vi "AI RT FIFO (by ref).vi"(0 "Data IN":dbl[](array[numeric]), 1 "Mode":T1=enum."Delete", 7 "Buffer Size":i32=10, 9 "# of elements":i32=1, 11 "Error IN":errorcluster, 12 "System Index":i32) -> (4 "Data OUT":dbl[][](array[numeric]), 6 "Empty?":bool, 8 "Size":i32, 15 "Error OUT":errorcluster)   [LabVIEW 2023]
uses:
  Type Defs and Controls/RT FIFO Mode.ctl
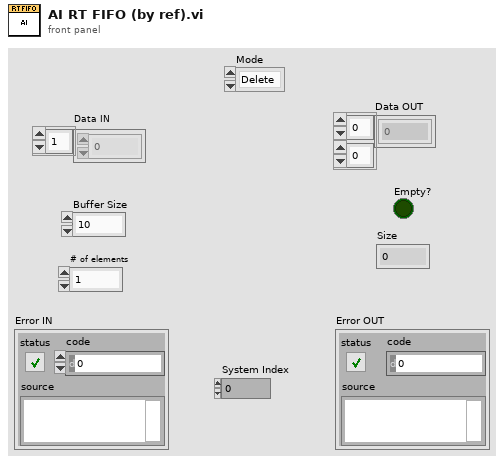
[diagram p1: front panel]
types:
  T1 = typedef "RT FIFO Mode.ctl" = enum16{"Create", "Write", "Read", "Delete"}
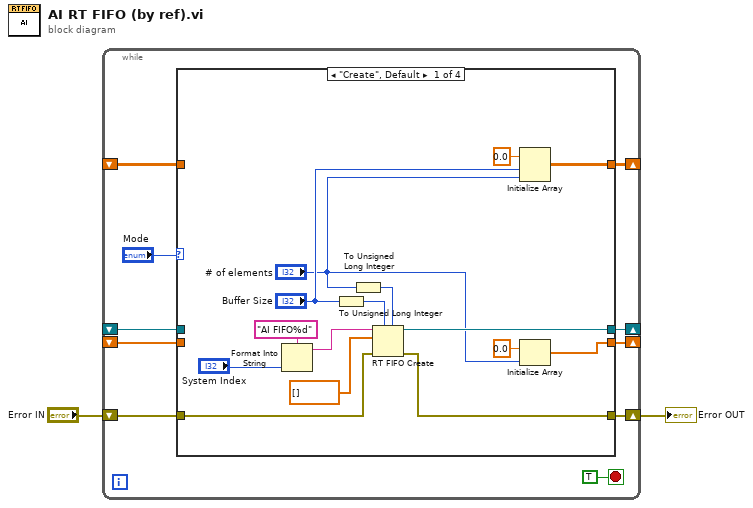
[diagram p0: block diagram]
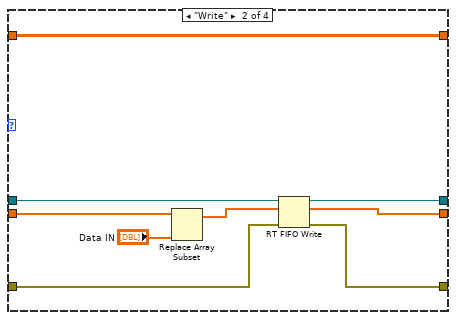
[diagram p2: hidden frame]
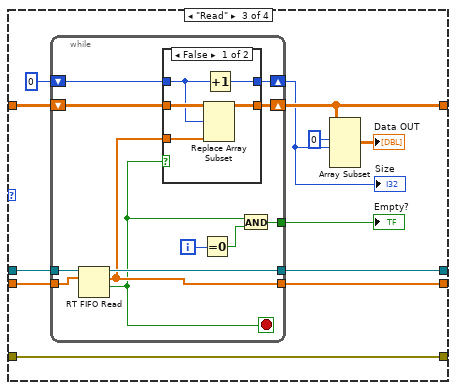
[diagram p3: hidden frame]
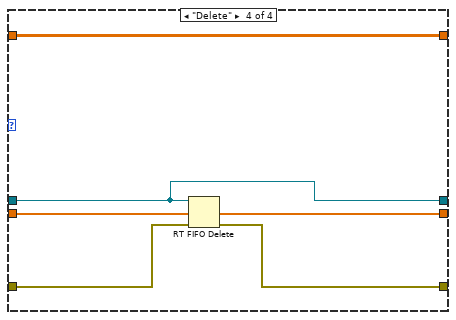
[diagram p5: hidden frame]
diagram:
  n1 = while {
    shift-right: [w10] -> _
    shift-left: _ -> [w9]
    shift-right: [w6] -> _
    shift-left: _ -> [w5]
    shift-right: [w4] -> _
    shift-left: _ -> [w3]
    shift-right: [w7] -> w1
    shift-left: "Error IN" -> [w8]
    stop <- TRUE stop-if-true
    n2 = case shown="\"Create\", Default" "Mode" {
      tunnel: [w27 w34 w45 w71] -> w10
      tunnel: w9 -> [_ w35 w46 w71]
      tunnel: w8 -> [w23 w30 w47 w69]
      tunnel: [w22 w29 w47 w68] -> w7
      tunnel: [w24 w31 w43 w70] -> w6
      tunnel: w5 -> [_ w33 w44 w70]
      tunnel: [w16 w28 w40 w67] -> w4
      tunnel: w3 -> [_ w28 w41 w67]
      frame "Create", Default {
        n3 = Format Into String(format string="AI FIFO%d" ("name (unnamed)"), "System Index") -> (resulting string=w13:string)  [unwired: 2 in, 1 out]
        n4 = To Unsigned Long Integer(number="Buffer Size") -> (unsigned 32bit integer=w17:u32)
        n5 = To Unsigned Long Integer(number="# of elements") -> (unsigned 32bit integer=w21:u32)
        n6 = RT FIFO Create(0:w13, 1:dbl[] [], 3:w23, 4:w17, 6:w21) -> (8:w27:refnum<k33>, 11:w22:errorcluster)  [unwired: 3 in, 1 out]
        n7 = Initialize Array(0.0, "Buffer Size", "# of elements") -> (w16:dbl[][])
        n8 = Initialize Array(0.0, "# of elements") -> (w24:dbl[])
      }
      frame "Write" {
        n9 = Replace Array Subset(array=w33, new element="Data IN") -> (w31:dbl[])  [unwired: 1 in]
        n10 = RT FIFO Write(0:w35, 1:w31, 3:w30) -> (8:w34:refnum<k33>, 11:w29:errorcluster)  [unwired: 2 in, 2 out]
      }
      frame "Read" {
        n11 = while {
          tunnel: w46 -> [w59]
          tunnel: [w58] -> w45
          tunnel: w44 -> [w57]
          tunnel: [w52] -> w43
          shift-right: [w55] -> w38
          shift-left: 0 -> [w56]
          shift-right: [w53] -> w40
          shift-left: w41 -> [w54]
          tunnel: [w48] -> w36
          i -> [w50]
          stop <- w51 stop-if-true
          n12 = RT FIFO Read(0:w59, 1:w57) -> (8:w58:refnum<k33>, 9:w52:dbl[], 10:w51:bool)  [unwired: 2 in, 2 out]
          n13 = case shown="False" w51 {
            tunnel: w56 -> [w61 w66]
            tunnel: [w64 w66] -> w55
            tunnel: w54 -> [w63 w65]
            tunnel: [w62 w65] -> w53
            tunnel: w52 -> [w60 _]
            frame False {
              n14 = Replace Array Subset(array=w63, new element=w60, index (row)=w61) -> (w62:dbl[][])  [unwired: 1 in]
              n15 = Increment(x=w61) -> (x+1=w64:i32)
            }
            frame True {
            }
          }
          n16 = Equal To 0?(x=w50) -> (x = 0?=w49:bool)
          n17 = And(x=w51, y=w49) -> (x .and. y?=w48:bool)
        }
        "Empty?" <- w36
        "Size" <- w38
        n18 = Array Subset(array=w40, index (row)=0 ("index"), length (row)=w38) -> (→"Data OUT":dbl[][])  [unwired: 2 in]
      }
      frame "Delete" {
        n19 = RT FIFO Delete(0:w71, 3:w69) -> (11:w68:errorcluster)  [unwired: 1 in]
      }
    }
  }
  "Error OUT" <- w1
